vi "lockDrive.vi"(9 "Steering Input":dbl, 10 "Throttle Input":dbl, 11 "Lock drive?":bool) -> (2 "Final Steering Value":dbl, 3 "Final Throttle Value":dbl, 7 "Boolean":bool)   [LabVIEW 2017]
uses:
  <vilib>/FRCT Team# 3937  Breakaway/Memory Library/memLib.lvlib
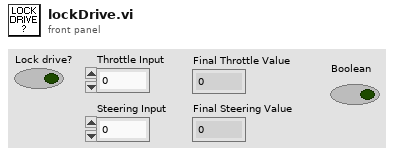
[diagram p1: front panel]
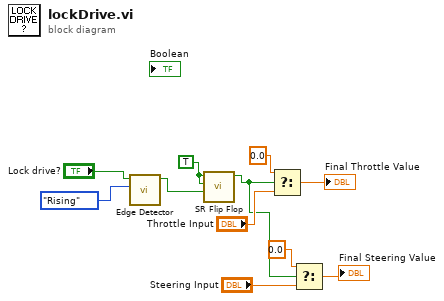
[diagram p0: block diagram]
diagram:
  w11 = TRUE ("Set")
  n1 = call <vilib>:"Edge Detector.vi"("Mode"=enum16{"Rising", "Falling", "Any"}."Rising", "Input"="Lock drive?") -> ("Output"=w10:bool)  [unwired: 9 in]
  n2 = call <vilib>:"SR Flip Flop.vi"("Enable"=w10, "Reset"=w11, "Set"=w11) -> ("Output"=w4:bool)  [unwired: 8 in]
  n3 = Select(t=0.0, s=w4, f="Throttle Input") -> (s? t:f=→"Final Throttle Value":dbl)
  n4 = Select(t=0.0, s=w4, f="Steering Input") -> (s? t:f=→"Final Steering Value":dbl)
